vi "Get Result.vi"(8 "error in (no error)":errorcluster, 11 "Ocean Optics Driver in":refnum<class "Ocean Optics Driver.lvclass">) -> (0 "error out":errorcluster, 2 "Result":refnum<class "Acquired Result.lvclass">, 3 "Ocean Optics Driver out":refnum<class "Ocean Optics Driver.lvclass">)   [LabVIEW 2016, in "Ocean Optics Driver.lvclass"]
uses:
  Ocean Optics Driver.lvclass
  <vilib>/express/express signal manip/GetorSetDDTAttributes/Set DDT Attributes/Set DDT Properties.xnode
  <vilib>/express/express shared/transition.llb/Dynamic To Waveform Array.vi
  <vilib>/express/express signal manip/GetorSetDDTAttributes/Set DDT Attributes/SetT0.vi
  <vilib>/express/express shared/transition.llb/Waveform Array To Dynamic.vi
  Spectrometer Driver/Spectrometer Driver.lvclass
  Results/Acquired Result/Acquired Result.lvclass
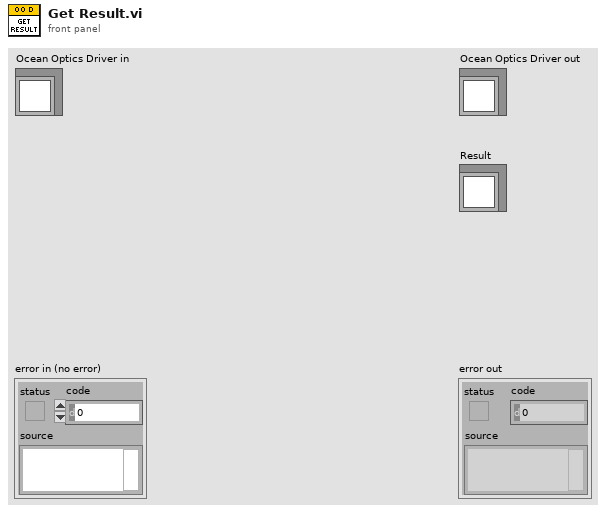
[diagram p1: front panel]
types:
  T1 = typedef "Ruby Spectra.lvclass/Ocean optics configuration.ctl" = cluster{"Integration time":dbl, "Fit parameters":T2, "Fit":bool, "Auto-update params":bool, "Save spectra":bool, "Reference wavelengh":dbl, "Background":path}
  T2 = typedef "Multi-peak Parameters.ctl" = cluster{"Function":enum16{"Gauss", "Lorentz"}, "Window width":dbl, "Initial guess":T3}
  T3 = typedef "Peak Parameters.ctl" = cluster{"Amplitude":dbl, "Center":dbl, "Width":dbl}
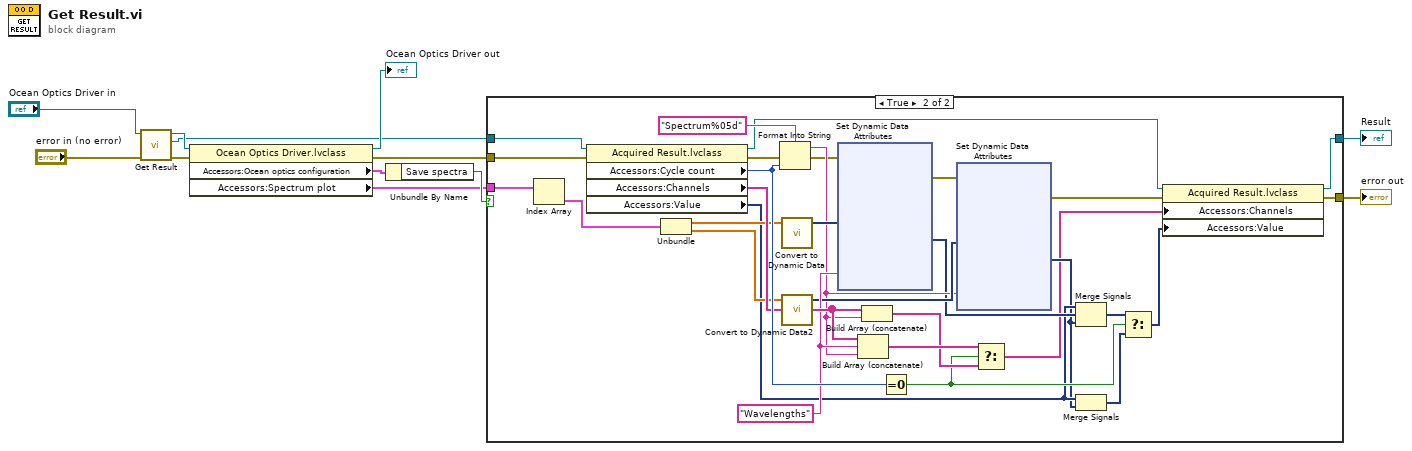
[diagram p0: block diagram]
diagram:
  n1 = call-parent "Get Result.vi"("error in (no error)"="error in (no error)", "Simple VISA Reader Driver in"="Ocean Optics Driver in") -> ("error out"=w12:errorcluster, "Result"=w5:refnum<class "Acquired Result.lvclass">, "Simple VISA Reader Driver out"=w9:refnum<class "Ocean Optics Driver.lvclass">)  [unwired: 7 in]
  n2 = property class="Ocean Optics Driver.lvclass"(reference=w9, error in=w12) -> (reference out=→"Ocean Optics Driver out":refnum<class "Ocean Optics Driver.lvclass">, error out=w4:errorcluster, "Accessors:Ocean optics configuration"=w7:T1, "Accessors:Spectrum plot"=w3:cluster{"Array":dbl[], "Array":dbl[]}[])
  n3 = Unbundle By Name(w7) -> ("Save spectra"=w6:bool)
  n4 = case shown="True" w6 {
    tunnel: w5 -> [w13 w44]
    tunnel: w4 -> [w14 w43]
    tunnel: w3 -> [_ w42]
    tunnel: [w14 w16] -> w1
    tunnel: [w13 w15] -> w2
    frame False {
    }
    frame True {
      w31 = "Wavelengths"
      n5 = Index Array(array=w42) -> (element=w41:cluster{"Array":dbl[], "Array":dbl[]})  [unwired: 1 in]
      n6 = property class="Acquired Result.lvclass"(reference=w44, error in=w43) -> (reference out=w22:refnum<class "Acquired Result.lvclass">, error out=w38:errorcluster, "Accessors:Cycle count"=w40:i32, "Accessors:Channels"=w35:string[], "Accessors:Value"=w26:dynamicdata)
      n7 = Unbundle(w41) -> ("Array"=w34:dbl[], "Array"=w33:dbl[])
      n8 = Format Into String(format string="Spectrum%05d", error in=w38, w40) -> (resulting string=w29:string, error out=w19:errorcluster)  [unwired: 1 in]
      n9 = call "Convert to Dynamic Data"("Array"=w34) -> ("Dynamic Data Type"=w32:dynamicdata)  [unwired: 3 in]
      n10 = call "Convert to Dynamic Data2"("Array"=w33) -> ("Dynamic Data Type"=w30:dynamicdata)  [unwired: 3 in]
      n11 = xnode "Set Dynamic Data Attributes"("Signals In"=w32, "Signal Name"=w31, "error in"=w19) -> ("Signals Out"=w27:dynamicdata, "error out"=w18:errorcluster)  [unwired: 1 in]
      n12 = Build Array (concatenate)(w35, w31, w29) -> (w37:string[])
      n13 = Build Array (concatenate)(w35, w29) -> (w36:string[])
      n14 = Equal To 0?(x=w40) -> (x = 0?=w28:bool)
      n15 = xnode "Set Dynamic Data Attributes"("Signals In"=w30, "Signal Name"=w29, "error in"=w18) -> ("Signals Out"=w25:dynamicdata, "error out"=w17:errorcluster)  [unwired: 1 in]
      n16 = Select(t=w37, s=w28, f=w36) -> (s? t:f=w21:string[])
      n17 = Merge Signals(w26, w27, w25) -> (w23:dynamicdata)
      n18 = Merge Signals(w26, w25) -> (w24:dynamicdata)
      n19 = Select(t=w23, s=w28, f=w24) -> (s? t:f=w20:dynamicdata)
      n20 = property class="Acquired Result.lvclass"(reference=w22, error in=w17, "Accessors:Channels"=w21, "Accessors:Value"=w20) -> (reference out=w15:refnum<class "Acquired Result.lvclass">, error out=w16:errorcluster)
    }
  }
  "error out" <- w1
  "Result" <- w2
